vi "file io array.vi"() -> ()   [LabVIEW 2012]
uses:
  <vilib>/Utility/file.llb/Write To Spreadsheet File (DBL).vi
  <vilib>/Utility/file.llb/Read From Spreadsheet File (DBL).vi
panel:
  out "all rows":dbl[][](array[numeric]) format="%0.3f"
  in  "Array":dbl[][](array[numeric])
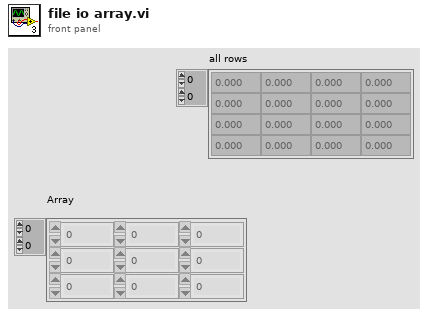
[diagram p1: front panel]
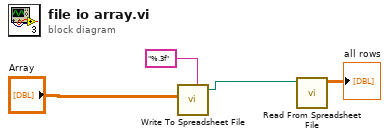
[diagram p0: block diagram]
diagram:
  n1 = call-poly <vilib>:"Write To Spreadsheet File.vi"("format (%.3f)"="%.3f", "2D data"="Array") -> ("new file path (Not A Path if cancelled)"=w2:path)  [unwired: 6 in]
  n2 = call-poly <vilib>:"Read From Spreadsheet File.vi"("file path (dialog if empty)"=w2) -> ("all rows"=→"all rows":dbl[][])  [unwired: 6 in, 4 out]
